vi "Test_Flux_Capacitor_GetAttributes.vi"(8 "error in (no error)":errorcluster, 10 "OnlyGetDvrReference(False)":bool, 11 "reference in":refnum<class "Test_Flux_Capacitor.lvclass">) -> (0 "error out":errorcluster, 1 "DataRef":refnum<data-value>, 2 "Data":T1, 3 "reference out":refnum<class "Test_Flux_Capacitor.lvclass">)   [LabVIEW 2022 SP3, in "Test_Flux_Capacitor.lvlib" / "Test_Flux_Capacitor.lvclass"]
uses:
  Test_Flux_Capacitor.lvclass
  protected/ObjectAttributes.ctl
  protected/Config.ctl
  Components/DMM_Keysight_34980A.lvlibp/DMM_Keysight_34980A.lvclass
  Components/LCR_BK891.lvlibp/LCR_BK891.lvclass
  Components/PSU_Base.lvlibp/PSU_Base.lvclass
  Components/SwitchBase.lvlibp/SwitchBase.lvclass
  Components/Flux_Capacitor.lvlibp/Flux_Capacitor.lvclass
  Components/Frequency_Counter_Base.lvlibp/Frequency_Counter_Base.lvclass
  Components/JTAG_Base.lvlibp/JTAG_Base.lvclass
  Test_Flux_Capacitor.lvclass/Test_Flux_Capacitor.ctl
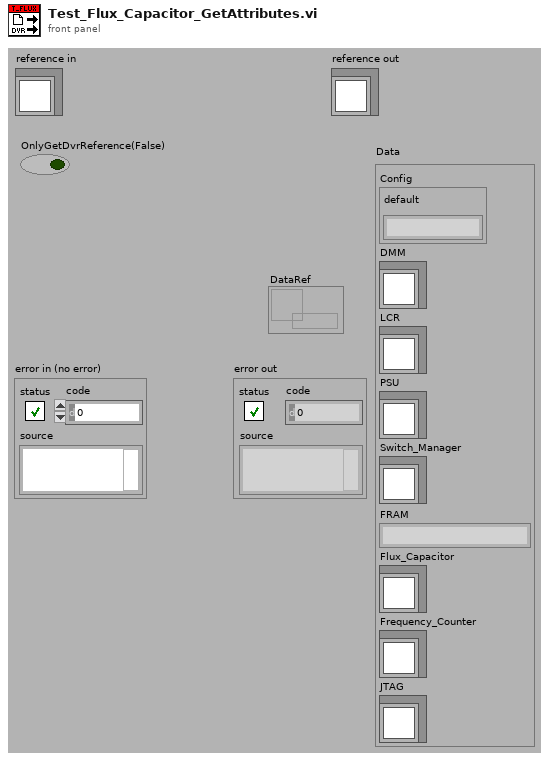
[diagram p1: front panel]
types:
  T1 = typedef "Test_Flux_Capacitor.lvlib/Test_Flux_Capacitor.lvclass/ObjectAttributes.ctl" = cluster{"Config":T2, "DMM":refnum<class "DMM_Keysight_34980A.lvclass">, "LCR":refnum<class "LCR_BK891.lvclass">, "PSU":refnum<class "PSU_Base.lvclass">, "Switch_Manager":refnum<class "SwitchBase.lvclass">, "FRAM":string, "Flux_Capacitor":refnum<class "Flux_Capacitor.lvclass">, "Frequency_Counter":refnum<class "Frequency_Counter_Base.lvclass">, "JTAG":refnum<class "JTAG_Base.lvclass">}
  T2 = typedef "Test_Flux_Capacitor.lvlib/Test_Flux_Capacitor.lvclass/Config.ctl" = cluster{"default":string}
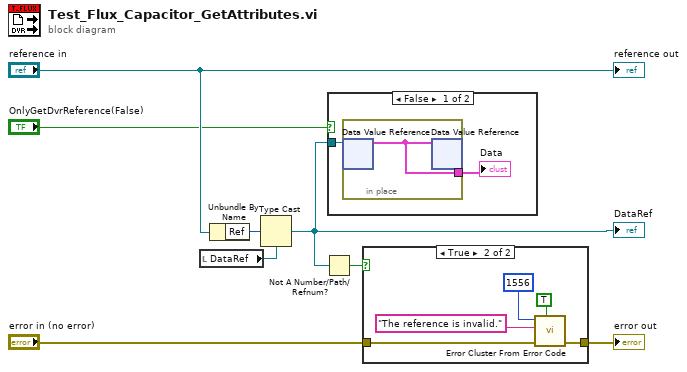
[diagram p0: block diagram]
diagram:
  n1 = local read "DataRef"() -> (w1:refnum<data-value>)
  n2 = Unbundle By Name("reference in") -> ("Ref"=w3:u32)
  n3 = Type Cast(type=w1, x=w3) -> (*(type *) &x=w5:refnum<data-value>)
  "DataRef" <- w5
  n4 = Not A Number/Path/Refnum?(number/path/refnum=w5) -> (NaN/Path/Refnum?=w2:bool)
  n5 = case shown="False" "OnlyGetDvrReference(False)" {
    tunnel: w5 -> [w10 _]
    frame False {
      n6 = in-place {
        in-place-border: [w11] -> w9
        n7 = in-place-dvr #1(w10) -> (w11:T1)  [unwired: 1 out]
        n8 = in-place-dvr #1(w11) -> ()  [unwired: 2 out]
      }
      "Data" <- w9
    }
    frame True {
    }
  }
  n9 = case shown="True" w2 {
    tunnel: "error in (no error)" -> [w12 w14]
    tunnel: [w12 w13] -> w7
    frame False {
    }
    frame True {
      n10 = call <vilib>:"Error Cluster From Error Code.vi"("show call chain? (False)"=TRUE, "error in (no error)"=w14, "error message (\"\")"="The reference is invalid." ("source"), "error code (0)"=1556 ("code")) -> ("error out"=w13:errorcluster)  [unwired: 5 in]
    }
  }
  "error out" <- w7
  "reference out" <- "reference in"
